vi "ziLVInit.vi"(8 "Error In":errorcluster) -> (0 "Error Out":errorcluster, 3 "ziHandle":T1 {"Handle" format="0x%08x"; "Conn" format="0x%08x"})   [LabVIEW 2009, in "Zurich Instruments LabOne.lvlib"]
doc: "Creates a connection to a ziLV API and loads dll into the memory"
uses:
  <instrlib>/Zurich Instruments LabOne/Zurich Instruments LabOne.lvlib
  <instrlib>/Zurich Instruments LabOne/Public/ziTypeHandle.ctl
  <vilib>/Utility/error.llb/DialogType.ctl
  <instrlib>/Zurich Instruments LabOne/Private/ziLV64.dll
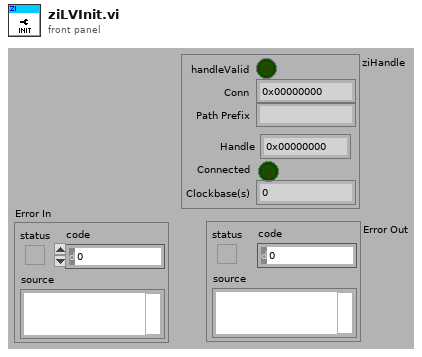
[diagram p1: front panel]
types:
  T1 = typedef "Zurich Instruments LabOne.lvlib/ziTypeHandle.ctl" = cluster{"handleValid":bool, "Conn":u64, "Path Prefix":string, "Handle":u64, "Connected":bool, "Clockbase(s)":dbl}
  T2 = typedef "DialogType.ctl" = u16
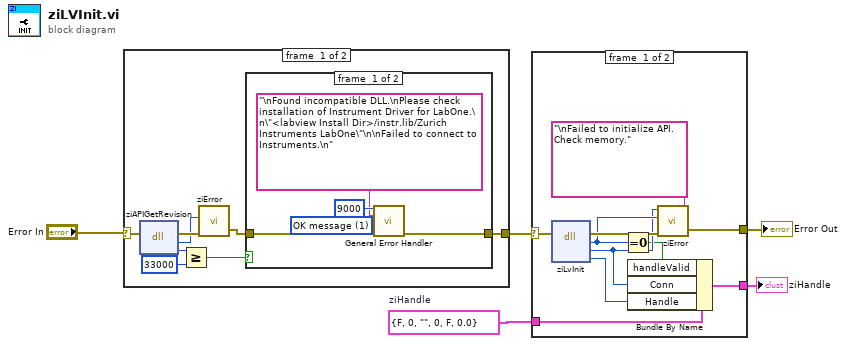
[diagram p0: block diagram]
diagram:
  w3 = T1 {"handleValid"=FALSE, "Conn"=0, "Path Prefix"="", "Handle"=0, "Connected"=FALSE, "Clockbase(s)"=0.0}  # ziHandle
  n1 = case shown="No Error" "Error In" {
    selector: "Error In" -> [w7 w20]
    tunnel: [w10 w20] -> w5
    frame #0 {
      n2 = dll-call lib="C:/Program Files/National Instruments/LabVIEW 2009/instr.lib/Zurich Instruments LabOne/Private/ziLV*.*" fn="ziAPIGetRevision" label="GetRev"(error in=w7) -> (error out=w9:errorcluster, "return type"=w8:u32, "rev"=w13:u32)  [unwired: 2 in, 2 out]
      n3 = Greater Or Equal?(x=w13, y=u32 33000 ("rev")) -> (x >= y?=w11:bool)
      n4 = call <instrlib>:"ziError.vi"("ziErrorCode"=w8, "Error In"=w9) -> ("Error Out"=w6:errorcluster)  [unwired: 4 in]
      n5 = case shown="False" w11 {
        tunnel: [w16 w19] -> w10
        tunnel: w6 -> [w18 w19]
        frame #0 {
          w17 = T2 1 items=["no dialog", "OK message", "continue or stop message", "OK message + warnings", "continue/stop + warnings"] ("type of dialog (OK msg:1)")
          n6 = call <vilib>:"General Error Handler.vi"("[error code] (0)"=9000, "[error source] (\" \")"="\nFound incompatible DLL.\nPlease check installation of Instrument Driver for LabOne.\n\"<labview Install Dir>/instr.lib/Zurich Instruments LabOne\"\n\nFailed to connect to Instruments.\n" ("message"), "type of dialog (OK msg:1)"=w17, "error in (no error)"=w18) -> ("error out"=w16:errorcluster)  [unwired: 7 in, 4 out]
        }
        frame #1 {
        }
      }
    }
    frame #1 {
    }
  }
  n7 = case shown="No Error" w5 {
    selector: w5 -> [w26 w32]
    tunnel: [w27 w32] -> w4
    tunnel: w3 -> [w22 w31]
    tunnel: [w21 w31] -> w1
    frame #0 {
      n8 = dll-call lib="C:/Program Files/National Instruments/LabVIEW 2009/instr.lib/Zurich Instruments LabOne/Private/ziLV*.*" fn="ziLvInit"(error in=w26) -> (error out=w30:errorcluster, "return type"=w28:u32, "Conn"=w24:u64, "ziLVHandle"=w25:u64)  [unwired: 2 in, 3 out]
      n9 = Equal To 0?(x=w28) -> (x = 0?=w23:bool)
      n10 = Bundle By Name(cluster=w22, "handleValid"=w23, "Conn"=w24, "Handle"=w25) -> (w21:T1)
      n11 = call <instrlib>:"ziError.vi"("Conn"=w24, "ziErrorCode"=w28, "Error In"=w30, "Annotation"="\nFailed to initialize API. Check memory." ("message")) -> ("Error Out"=w27:errorcluster)  [unwired: 2 in]
    }
    frame #1 {
    }
  }
  "Error Out" <- w4
  "ziHandle" <- w1
